vi "Initialize Configuration.vi"(8 "error in (no error)":errorcluster, 11 "Instrument in":refnum<class "Instrument.lvclass">) -> (0 "error out":errorcluster, 3 "Instrument out":refnum<class "Instrument.lvclass">)   [LabVIEW 2019, in "Instrument.lvclass"]
uses:
  Instrument.lvclass
  Instrument.lvclass/Instrument.ctl
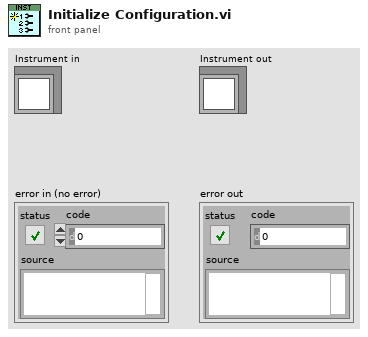
[diagram p1: front panel]
types:
  T1 = typedef "RemoteControl.lvclass/RC Com Type--enum.ctl" = enum16{"RC", "STM", "ZMQ"}
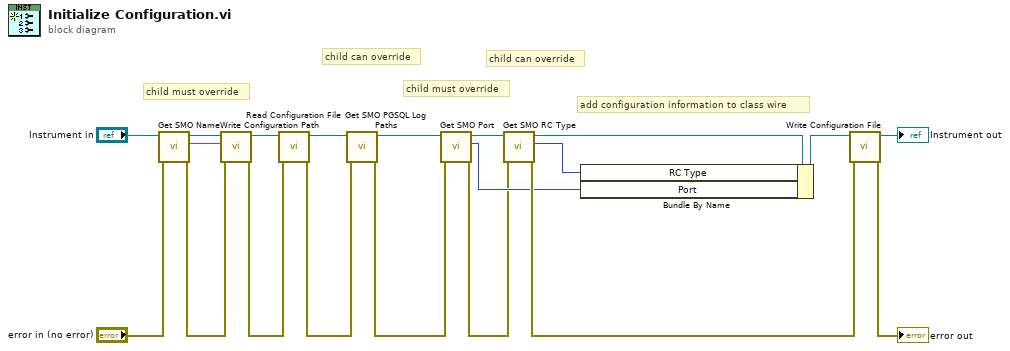
[diagram p0: block diagram]
diagram:
  # "child can override"
  # "child can override"
  # "child must override"
  # "child must override"
  # "add configuration information to class wire"
  n1 = call-dynamic "Get SMO Name.vi"("error in (no error)"="error in (no error)", "Instrument in"="Instrument in") -> ("error out"=w3:errorcluster, "SMO Name"=w16:string, "Instrument out"=w4:refnum<class "Instrument.lvclass">)  [unwired: 7 in]
  n2 = call "Write Configuration Path.vi"("error in (no error)"=w3, "name or relative path"=w16, "Instrument in"=w4) -> ("error out"=w11:errorcluster, "Instrument out"=w10:refnum<class "Instrument.lvclass">)  [unwired: 7 in]
  n3 = call-dynamic "Read Configuration File.vi"("error in (no error)"=w11, "Instrument in"=w10) -> ("error out"=w14:errorcluster, "Instrument out"=w12:refnum<class "Instrument.lvclass">)  [unwired: 8 in]
  n4 = call-dynamic "Get SMO PGSQL Log Paths.vi"("error in (no error)"=w14, "Instrument in"=w12) -> ("error out"=w15:errorcluster, "Instrument out"=w13:refnum<class "Instrument.lvclass">)  [unwired: 7 in, 1 out]
  n5 = call-dynamic "Get SMO Port.vi"("error in (no error)"=w15, "Instrument in"=w13) -> ("error out"=w7:errorcluster, "Port"=w8:u16, "Instrument out"=w5:refnum<class "Instrument.lvclass">)  [unwired: 7 in]
  n6 = call-dynamic "Get SMO RC Type.vi"("error in (no error)"=w7, "Instrument in"=w5) -> ("error out"=w18:errorcluster, "RC Type"=w6:T1, "Instrument out"=w9:refnum<class "Instrument.lvclass">)  [unwired: 7 in]
  n7 = Bundle By Name(cluster=w9, "RC Type"=w6, "Port"=w8) -> (w20:refnum<class "Instrument.lvclass">)
  n8 = call-dynamic "Write Configuration File.vi"("error in (no error)"=w18, "Instrument in"=w20) -> ("error out"=→"error out":errorcluster, "Instrument out"=→"Instrument out":refnum<class "Instrument.lvclass">)  [unwired: 8 in]
